vi "get file name and extension from path.vi"(11 "fiel path":path) -> (1 "file extension":string, 3 "file name":string, 5 "folder path":path)   [LabVIEW 2023, in "File Classes.lvlib"]
uses:
  File Classes.lvlib
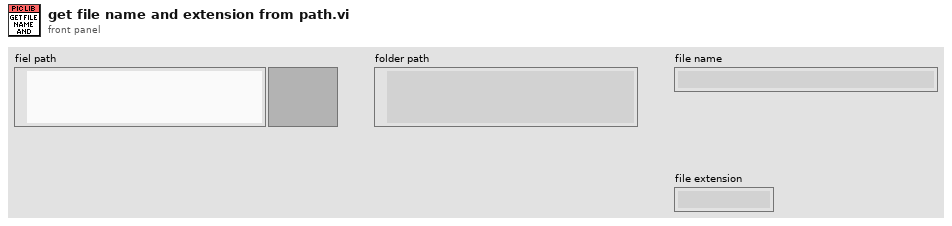
[diagram p1: front panel]
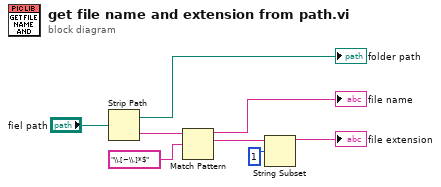
[diagram p0: block diagram]
diagram:
  n1 = Strip Path(path="fiel path") -> (stripped path=→"folder path":path, name=w3:string)
  n2 = Match Pattern(string=w3, regular expression="\\.[~\\.]*$") -> (before substring=→"file name":string, match substring=w7:string)  [unwired: 3 out]
  n3 = String Subset(string=w7, offset (0)=1) -> (substring=→"file extension":string)  [unwired: 1 out]
